vi "Get Open batch .vi"(8 "error in (no error) 5":errorcluster, 11 "Module Number  2":dbl=1.0) -> (0 "error out":errorcluster, 3 "subarray":string[](array[string]))   [LabVIEW 2015, in "Copy of Untitled Library 1.lvlib"]
uses:
  Copy of Untitled Library 1.lvlib
  Controls/Enum Constant.ctl
  <userlib>/origin_lib_main/db_interface/DB Operations Enum.ctl
  <vilib>/addons/database/_DB Variant To Data/Database Variant To Data.xnode
  <userlib>/origin_lib_main/db_interface/DB Interface.lvlib
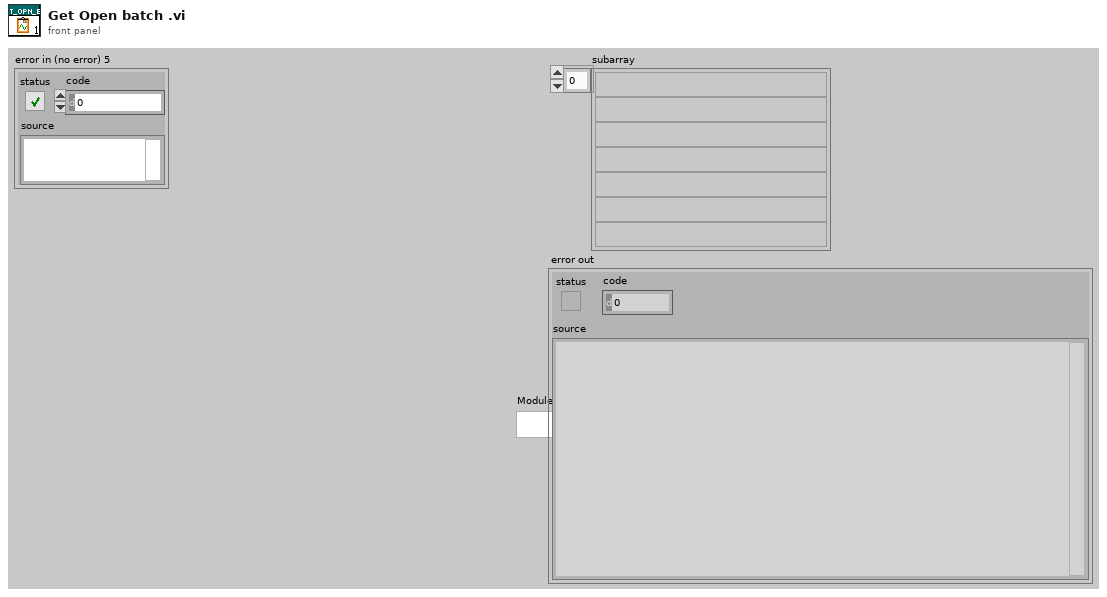
[diagram p1: front panel]
types:
  T1 = typedef "DB Interface.lvlib/DB Operations Enum.ctl" = enum16{"Select", "Update", "Insert", "Delete", "Fetch SQL Query", "Execute SQL Query", "Drop Table", "List Tables"}
  T2 = typedef "Enum Constant.ctl" = enum16{"Init", "Read", "Write"}
  T3 = typedef "FGV Data.ctl" = T4[]
  T4 = typedef "FGV Cluster Data.ctl" = cluster{"Manual/Automatic":bool, "UI Controllers ":string[], "UI Primery Key ":dbl[], "Caller Queue & MSG":T5, "Module ID":dbl, "DB Reference In":T6, "Products Columns":string[], "Cluster":cluster{"Delete Product":enum8{"Enabled", "Disabled", "Disabled and Grayed Out"}, "Add Product ":enum8{"Enabled", "Disabled", "Disabled and Grayed Out"}, "EDIT BATCH":enum8{"Enabled", "Disabled", "Disabled and Grayed Out"}, "Open Batch ":enum8{"Enabled", "Disabled", "Disabled and Grayed Out"}, "Close Batch":enum8{"Enabled", "Disabled", "Disabled and Grayed Out"}, "Delete Batch":enum8{"Enabled", "Disabled", "Disabled and Grayed Out"}, "Add Batch ":enum8{"Enabled", "Disabled", "Disabled and Grayed Out"}}}
  T5 = typedef "Queue and Caller MSG.ctl" = cluster{"Caller Queue":refnum<queue>, "Caller MSG":string}
  T6 = typedef "NI_Database_API.lvlib/Conn ObjectReference.ctl" = refnum<k1>
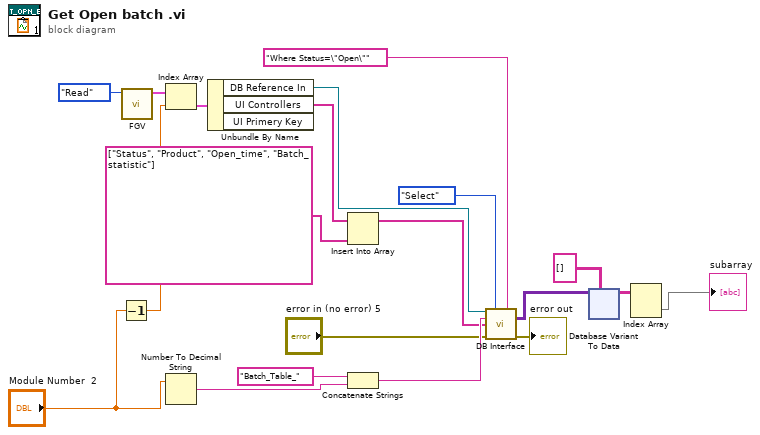
[diagram p0: block diagram]
diagram:
  n1 = Decrement(x="Module Number  2") -> (x-1=w13:dbl)
  n2 = call "FGV.vi"("Enum"=Enum_Constant."Read") -> ("Read Data"=w15:T3)  [unwired: 9 in, 1 out]
  n3 = Index Array(array=w15, index=w13) -> (element=w14:T4)
  n4 = Number To Decimal String(number="Module Number  2") -> (decimal integer string=w17:string)  [unwired: 1 in]
  n5 = Unbundle By Name(w14) -> ("DB Reference In"=w8:T6, "UI Controllers"=w7:string[])  [unwired: 1 out]
  n6 = Insert Into Array(array=w7, new element=string[] ["Status", "Product", "Open_time", "Batch_statistic"] ("element")) -> (w4:string[])  [unwired: 1 in]
  n7 = Concatenate Strings("Batch_Table_" ("string"), w17) -> (w16:string)
  n8 = call <userlib>:"DB Interface.vi"("DB Ref In"=w8, "Operation"=DB_Operations_Enum."Select", "condition"="Where Status=\"Open\"", "DB Table"=w16, "DB columns"=w4, "error in (no error)"="error in (no error) 5") -> ("data Out"=w10:variant[][], "error out"=→"error out":errorcluster)  [unwired: 6 in, 2 out]
  n9 = xnode "Database Variant To Data"("database variant"=w10, "type"=string[][] [] ("columns")) -> ("data"=w11:string[][])  [unwired: 1 in, 1 out]
  n10 = Index Array(array=w11) -> (element=→"subarray":string[])  [unwired: 2 in]
